vi "SequenceRun.vi"(5 "EndTime":timestamp, 7 "StartTime":timestamp, 8 "error in":errorcluster, 11 "OperationRun":refnum<class "SequenceRun.lvclass">) -> (0 "error out":errorcluster, 3 "Passed":bool)   [LabVIEW 2020]
uses:
  <vilib>/Averna/ProligentResultProcessor/ProligentResultProcessor.lvlibp/SequenceRun/SequenceRun/SequenceRun.lvclass
  <vilib>/Averna/ProligentResultProcessor/ProligentResultProcessor.lvlibp/SequenceRun/SequenceRun/SetSequenceFullName.vi
  <vilib>/Averna/ProligentResultProcessor/ProligentResultProcessor.lvlibp/SequenceRun/SequenceRun/SetStationFullName.vi
  <vilib>/Averna/ProligentResultProcessor/ProligentResultProcessor.lvlibp/SequenceRun/SequenceRun/SetStartDate.vi
  <vilib>/Averna/ProligentResultProcessor/ProligentResultProcessor.lvlibp/SequenceRun/SequenceRun/SetSequenceExecutionStatus.vi
  <vilib>/Averna/ProligentResultProcessor/ProligentResultProcessor.lvlibp/SequenceRun/SequenceRun/SetEndDate.vi
  <vilib>/Averna/ProligentResultProcessor/ProligentResultProcessor.lvlibp/SequenceRun/SequenceRun/SetSequenceRunId.vi
  <vilib>/Averna/ProligentResultProcessor/ProligentResultProcessor.lvlibp/SequenceRun/SequenceRun/SetSequenceVersion.vi
  <vilib>/Averna/ProligentResultProcessor/ProligentResultProcessor.lvlibp/SequenceRun/SequenceRun/GetUser.vi
  <vilib>/Averna/ProligentResultProcessor/ProligentResultProcessor.lvlibp/SequenceRun/SequenceRun/GetSequenceFullName.vi
  <vilib>/Averna/ProligentResultProcessor/ProligentResultProcessor.lvlibp/SequenceRun/SequenceRun/GetStationFullName.vi
  <vilib>/Averna/ProligentResultProcessor/ProligentResultProcessor.lvlibp/SequenceRun/SequenceRun/GetStartDate.vi
  <vilib>/Averna/ProligentResultProcessor/ProligentResultProcessor.lvlibp/SequenceRun/SequenceRun/GetSequenceExecutionStatus.vi
  <vilib>/Averna/ProligentResultProcessor/ProligentResultProcessor.lvlibp/SequenceRun/SequenceRun/GetEndDate.vi
  <vilib>/Averna/ProligentResultProcessor/ProligentResultProcessor.lvlibp/SequenceRun/SequenceRun/GetSequenceRunId.vi
  <vilib>/Averna/ProligentResultProcessor/ProligentResultProcessor.lvlibp/SequenceRun/SequenceRun/GetSequenceVersion.vi
  <vilib>/Averna/ProligentResultProcessor/ProligentResultProcessor.lvlibp/SequenceRun/SequenceRun/GetStepRuns.vi
  <vilib>/Averna/ProligentResultProcessor/ProligentResultProcessor.lvlibp/SequenceRun/SequenceRun/GetCharacteristics.vi
  <vilib>/Averna/ProligentResultProcessor/ProligentResultProcessor.lvlibp/SequenceRun/SequenceRun/GetDocuments.vi
  <vilib>/Averna/ProligentResultProcessor/ProligentResultProcessor.lvlibp/SequenceRun/SequenceRun/GetFailureReferences.vi
  <vilib>/Averna/ProligentResultProcessor/ProligentResultProcessor.lvlibp/SequenceRun/SequenceRun/GetCustomData.vi
  <vilib>/Averna/ProligentResultProcessor/ProligentResultProcessor.lvlibp/StepRun/StepRun/StepRun.lvclass
  <vilib>/Averna/ProligentResultProcessor/ProligentResultProcessor.lvlibp/Model/Characteristic/Characteristic.lvclass
  <vilib>/Averna/ProligentResultProcessor/ProligentResultProcessor.lvlibp/Model/Document/Document.lvclass
  <vilib>/Averna/ProligentResultProcessor/ProligentResultProcessor.lvlibp/Failure/FailureReference/FailureReference.lvclass
  <vilib>/Averna/ProligentResultProcessor/ProligentResultProcessor.lvlibp/Model/CustomData/CustomData.lvclass
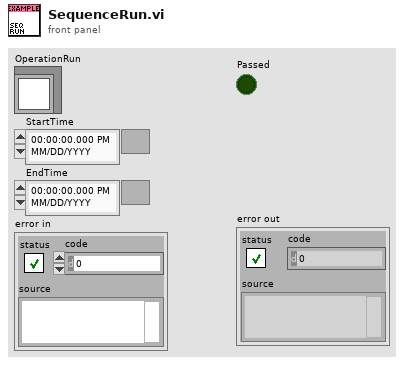
[diagram p1: front panel]
types:
  T1 = enum16{"PASS", "FAIL", "NOT_COMPLETED", "ABORTED"}
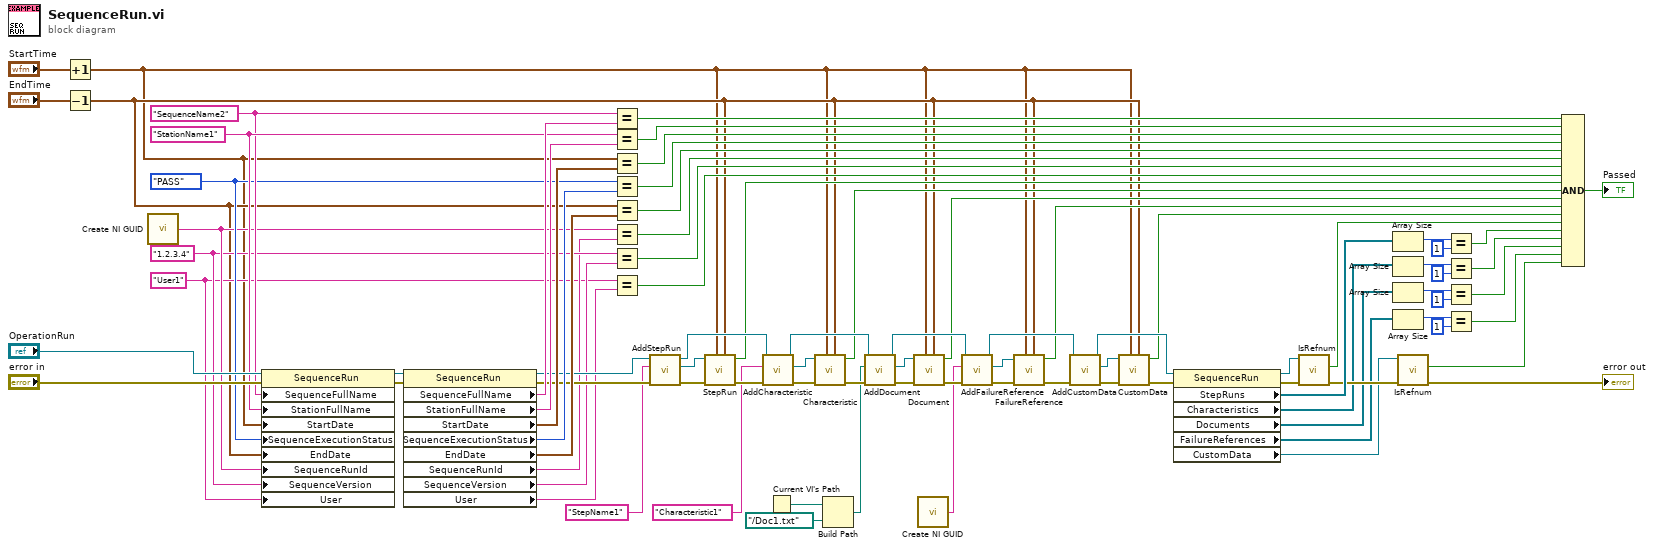
[diagram p0: block diagram]
diagram:
  w3 = "User1"
  w13 = "1.2.3.4"
  w63 = T1."PASS" ("ProcessRunStatus")
  w78 = "StationName1"
  w77 = "SequenceName2"
  n1 = Increment(x="StartTime") -> (x+1=w1:timestamp)
  n2 = Decrement(x="EndTime") -> (x-1=w2:timestamp)
  n3 = call <vilib>:"Create NI GUID.vi"() -> ("NI GUID"=w14:string)
  n4 = property class="SequenceRun"(reference="OperationRun", error in="error in", "SequenceFullName"=w77, "StationFullName"=w78, "StartDate"=w1, "SequenceExecutionStatus"=w63, "EndDate"=w2, "SequenceRunId"=w14, "SequenceVersion"=w13, "User"=w3) -> (reference out=w85:refnum<class "SequenceRun.lvclass">, error out=w84:errorcluster)
  n5 = property class="SequenceRun"(reference=w85, error in=w84) -> (reference out=w76:refnum<class "SequenceRun.lvclass">, error out=w75:errorcluster, "SequenceFullName"=w83:string, "StationFullName"=w82:string, "StartDate"=w81:timestamp, "SequenceExecutionStatus"=w80:T1, "EndDate"=w79:timestamp, "SequenceRunId"=w11:string, "SequenceVersion"=w12:string, "User"=w5:string)
  n6 = Equal?(x=w77, y=w83) -> (x = y?=w70:bool)
  n7 = Equal?(x=w78, y=w82) -> (x = y?=w69:bool)
  n8 = Equal?(x=w1, y=w81) -> (x = y?=w68:bool)
  n9 = Equal?(x=w63, y=w80) -> (x = y?=w67:bool)
  n10 = Equal?(x=w2, y=w79) -> (x = y?=w66:bool)
  n11 = Equal?(x=w14, y=w11) -> (x = y?=w10:bool)
  n12 = Equal?(x=w13, y=w12) -> (x = y?=w9:bool)
  n13 = Equal?(x=w3, y=w5) -> (x = y?=w4:bool)
  n14 = call <vilib>:"AddStepRun.vi"("error in"=w75, "StepName"="StepName1", "SequenceRun in"=w76) -> ("error out"=w58:errorcluster, "StepRun"=w57:refnum<class "StepRun.lvclass">, "SequenceRun out"=w59:refnum<class "SequenceRun.lvclass">)  [unwired: 6 in]
  n15 = call "StepRun.vi"("EndTime"=w2, "StartTime"=w1, "error in"=w58, "StepRun"=w57) -> ("error out"=w52:errorcluster, "Passed"=w40:bool)  [unwired: 6 in]
  n16 = call <vilib>:"AddCharacteristic.vi"("error in"=w52, "FullName"="Characteristic1", "SequenceRun in"=w59) -> ("error out"=w51:errorcluster, "Characteristic"=w50:refnum<class "Characteristic.lvclass">, "SequenceRun out"=w53:refnum<class "SequenceRun.lvclass">)  [unwired: 6 in]
  n17 = Current VI's Path() -> (path=w8:path)
  n18 = call "Characteristic.vi"("EndTime"=w2, "StartTime"=w1, "error in (no error)"=w51, "Characteristic in"=w50) -> ("error out"=w47:errorcluster, "Passed"=w39:bool)  [unwired: 6 in]
  n19 = Build Path(base path=w8, name or relative path=path "../Doc1.txt") -> (appended path=w6:path)
  n20 = call <vilib>:"AddDocument.vi"("error in"=w47, "FilePath"=w6, "SequenceRun in"=w53) -> ("error out"=w46:errorcluster, "Document"=w45:refnum<class "Document.lvclass">, "SequenceRun out"=w48:refnum<class "SequenceRun.lvclass">)  [unwired: 6 in]
  n21 = call "Document.vi"("EndTime"=w2, "StartTime"=w1, "error in (no error)"=w46, "Document in"=w45) -> ("error out"=w43:errorcluster, "Passed"=w38:bool)  [unwired: 6 in]
  n22 = call <vilib>:"Create NI GUID.vi"() -> ("NI GUID"=w16:string)
  n23 = call <vilib>:"AddFailureReference.vi"("error in"=w43, "Id"=w16, "SequenceRun in"=w48) -> ("error out"=w42:errorcluster, "Document"=w41:refnum<class "FailureReference.lvclass">, "SequenceRun out"=w44:refnum<class "SequenceRun.lvclass">)  [unwired: 6 in]
  n24 = call "FailureReference.vi"("EndTime"=w2, "StartTime"=w1, "error in"=w42, "FailureReference"=w41) -> ("error out"=w35:errorcluster, "Passed"=w37:bool)  [unwired: 6 in]
  n25 = call <vilib>:"AddCustomData.vi"("error in"=w35, "SequenceRun in"=w44) -> ("error out"=w34:errorcluster, "CustomData"=w32:refnum<class "CustomData.lvclass">, "SequenceRun out"=w36:refnum<class "SequenceRun.lvclass">)  [unwired: 7 in]
  n26 = call "CustomData.vi"("EndTime"=w2, "StartTime"=w1, "error in"=w34, "CustomData"=w32) -> ("error out"=w33:errorcluster, "Passed"=w15:bool)  [unwired: 6 in]
  n27 = property class="SequenceRun"(reference=w36, error in=w33) -> (reference out=w55:refnum<class "SequenceRun.lvclass">, error out=w71:errorcluster, "StepRuns"=w72:refnum<class "StepRun.lvclass">[], "Characteristics"=w25:refnum<class "Characteristic.lvclass">[], "Documents"=w24:refnum<class "Document.lvclass">[], "FailureReferences"=w23:refnum<class "FailureReference.lvclass">[], "CustomData"=w18:refnum<class "CustomData.lvclass">)
  n28 = call <vilib>:"IsRefnum.vi"("error in"=w71, "SequenceRun in"=w55) -> ("error out"=w56:errorcluster, "IsRefnum"=w54:bool)  [unwired: 7 in, 1 out]
  n29 = Array Size(array=w72) -> (size(s)=w74:i32)
  n30 = Array Size(array=w25) -> (size(s)=w30:i32)
  n31 = Array Size(array=w24) -> (size(s)=w29:i32)
  n32 = Array Size(array=w23) -> (size(s)=w26:i32)
  n33 = call <vilib>:"IsRefnum.vi"("error in"=w56, "CustomDataType in"=w18) -> ("error out"=→"error out":errorcluster, "IsRefnum"=w17:bool)  [unwired: 7 in, 1 out]
  n34 = Equal?(x=w74, y=1) -> (x = y?=w65:bool)
  n35 = Equal?(x=w30, y=1) -> (x = y?=w22:bool)
  n36 = Equal?(x=w29, y=1) -> (x = y?=w21:bool)
  n37 = Equal?(x=w26, y=1) -> (x = y?=w20:bool)
  n38 = Compound Arithmetic op=AND(w70, w69, w68, w67, w66, w10, w9, w4, w40, w39, w38, w37, w15, w54, w65, w22, w21, w20, w17) -> (→"Passed":bool)
